vi "Exit.vi"(8 "error in":errorcluster, 11 "Notifiers":T1) -> (0 "error out":errorcluster)   [LabVIEW 2014, in "Model.lvlib"]
uses:
  Model.lvlib
  support/Message Queue/Message Queue.lvlib
  Support/Notifiers/Notifiers.ctl
  Support/Notifiers/Notifiers.lvlib
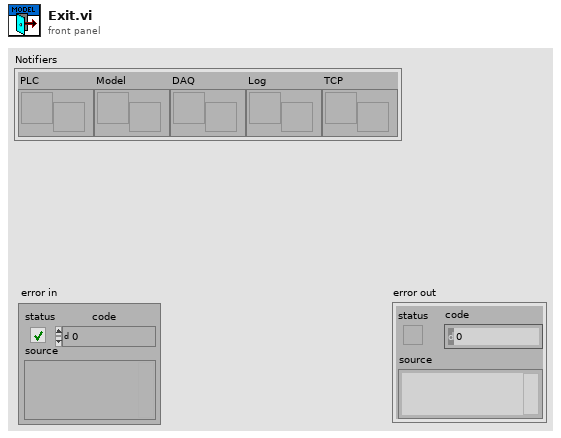
[diagram p1: front panel]
types:
  T1 = typedef "Notifiers.lvlib/Notifiers.ctl" = cluster{"PLC":refnum<notifier>, "Model":refnum<notifier>, "DAQ":refnum<notifier>, "Log":refnum<notifier>, "TCP":refnum<notifier>}
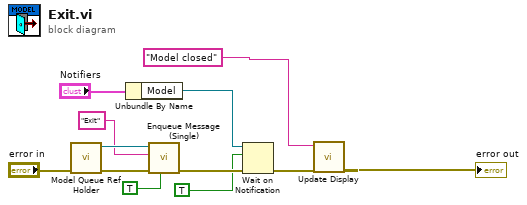
[diagram p0: block diagram]
diagram:
  n1 = call "Model Queue Ref Holder.vi"("error in"="error in") -> ("error out"=w12:errorcluster, "Input Message Queue"=w10:refnum<queue>)  [unwired: 9 in]
  n2 = Unbundle By Name("Notifiers") -> ("Model"=w5:refnum<notifier>)
  n3 = call "Enqueue Message (Single).vi"("Priority Message? (F)"=TRUE, "error in (no error)"=w12, "Message"="Exit", "Message Queue"=w10) -> ("error out"=w8:errorcluster)  [unwired: 6 in, 1 out]
  n4 = Wait on Notification(notifier=w5, ignore previous (F)=TRUE, error in (no error)=w8) -> (error out=w4:errorcluster)  [unwired: 1 in, 3 out]
  n5 = call "Update Display.vi"("error in"=w4, "Message string"="Model closed" ("Message")) -> ("error out"=→"error out":errorcluster)  [unwired: 9 in]
